vi "CallDaqMeasure.vi"(8 "error in (no error)":errorcluster, 11 "TopUI in":refnum<class "TopUI.lvclass">) -> (0 "error out":errorcluster, 3 "TopUI out":refnum<class "TopUI.lvclass">)   [LabVIEW 2020, in "TopUI.lvlib" / "TopUI.lvclass"]
uses:
  TopUI.lvclass
  SimDaq/SimDaq Messages/Measure Msg/Measure Msg.lvclass
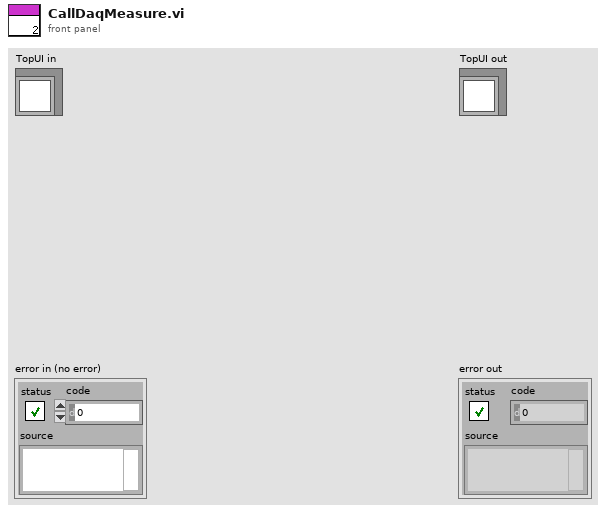
[diagram p1: front panel]
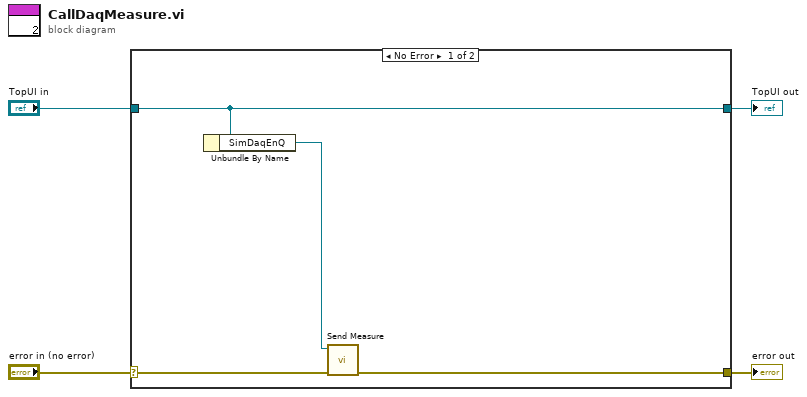
[diagram p0: block diagram]
diagram:
  n1 = case shown="No Error" "error in (no error)" {
    selector: "error in (no error)" -> [w8 w10]
    tunnel: [w6 w10] -> w3
    tunnel: [w7 w9] -> w1
    tunnel: "TopUI in" -> [w7 w9]
    frame No Error {
      n2 = Unbundle By Name(w7) -> ("SimDaqEnQ"=w5:refnum<class "Message Enqueuer.lvclass">)
      n3 = call "Send Measure.vi"("error in (no error)"=w8, "Message Enqueuer"=w5) -> ("error out"=w6:errorcluster)  [unwired: 8 in, 1 out]
    }
    frame Error {
    }
  }
  "error out" <- w3
  "TopUI out" <- w1
